vi "MPUSBWrite.vi"(6 "dwMilliseconds":u32=1000, 8 "error in (no error)":errorcluster, 9 "pDataIn":u8[](array[numeric]), 10 "dwLen":u32, 11 "handleIn":u32 format="%x") -> (0 "error out":errorcluster, 1 "pDataOut":u8[](array[numeric]), 2 "return type":u32, 3 "handleOut":u32 format="%x", 5 "pLength (out)":u32)   [LabVIEW 2016]
doc: "// Note that \"input\" and \"output\" refer to the parameter designations in calls\n// to this function, which are the opposite of common sense from the\n// perspective of an application making the calls.\n//\nDWORD MPUSBWrite(HANDLE handle, // Input\n PVOID pData, // Input\n DWORD dwLen, // Input\n PDWORD pLength, // Output\n DWORD dwMilliseconds); // Input\n\nWritten by: Complete Automated Solutions\nwww.CompleteAutomatedSolutions.com"
uses:
  Documents/Software/EPR DAQ/qsm/trunk/Hardware/Firgelli/USB_VIs/mpusbapi.dll
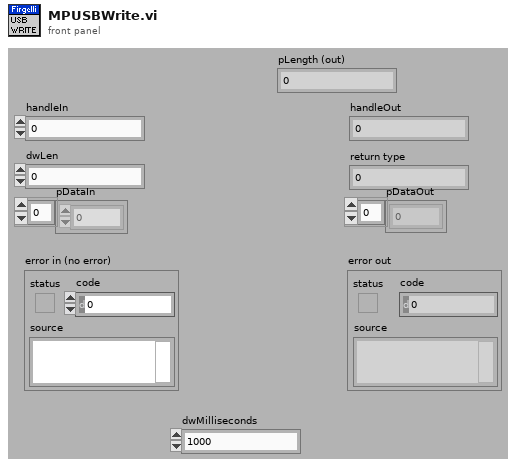
[diagram p1: front panel]
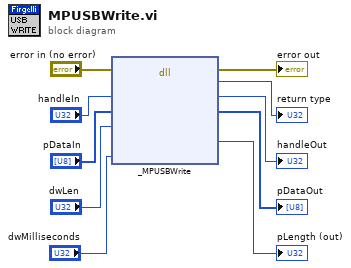
[diagram p0: block diagram]
diagram:
  n1 = dll-call lib="C:/Users/Wilson Schreiber/Documents/Software/EPR DAQ/qsm/trunk/Hardware/Firgelli/USB_VIs/mpusbapi.dll" fn="_MPUSBWrite"(error in="error in (no error)", "handle"="handleIn", "pData"="pDataIn", "dwLen"="dwLen", "dwMilliseconds"="dwMilliseconds") -> (error out=→"error out":errorcluster, "return type"=→"return type":u32, "handle"=→"handleOut":u32, "pData"=→"pDataOut":u8[], "pLength"=→"pLength (out)":u32)  [unwired: 4 in, 2 out]
